vi "length 2 dlc.vi"(1 "length":i32) -> (0 "dlc":u8)   [LabVIEW 2024, in "atsj peakcan basic.lvlib"]
uses:
  atsj peakcan basic.lvlib
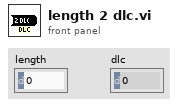
[diagram p1: front panel]
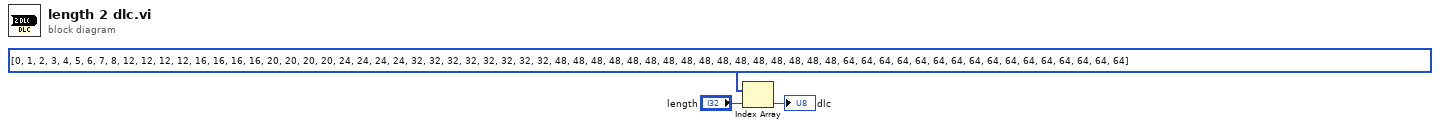
[diagram p0: block diagram]
diagram:
  n1 = Index Array(array=u8[] [0, 1, 2, 3, 4, 5, 6, 7, 8, 12, 12, 12, 12, 16, 16, 16, 16, 20, 20, 20, 20, 24, 24, 24, 24, 32, 32, 32, 32, 32, 32, 32, 32, 48, 48, 48, 48, 48, 48, 48, 48, 48, 48, 48, 48, 48, 48, 48, 48, 64, 64, 64, 64, 64, 64, 64, 64, 64, 64, 64, 64, 64, 64, 64, 64] ("Array"), index="length") -> (element=→"dlc":u8)
